vi "SendPanelUIReference.vi"(8 "error in (no error)":errorcluster, 10 "VI Refnum":refnum<vi>, 11 "Device in":refnum<class "Device.lvclass">) -> (0 "error out":errorcluster, 3 "Device out":refnum<class "Device.lvclass">)   [LabVIEW 2020, in "Device.lvlib" / "Device.lvclass"]
uses:
  Device.lvclass
  C:/Program Files/National Instruments/LabVIEW 2020/vi.lib/ActorFramework/Actor/Actor.lvclass
  <vilib>/ActorFramework/Actor/Actor.lvclass/Actor.ctl
  Interface/Communication Messages/Send Panel Refercence Msg/Send Panel Refercence Msg.lvclass/Send Panel Refercence Msg.ctl
  <vilib>/ActorFramework/Message Enqueuer/Message Enqueuer.lvclass/Message Enqueuer.ctl
  <vilib>/ActorFramework/Message Enqueuer/Enqueue.vi
  Interface/Communication Messages/Send Panel Refercence Msg/Send Panel Refercence Msg.lvclass
  C:/Program Files/National Instruments/LabVIEW 2020/vi.lib/ActorFramework/Message/Message.lvclass
  <vilib>/ActorFramework/Message Priority Queue/Priority Enqueue.vi
  <vilib>/ActorFramework/Actor/Actor.lvclass
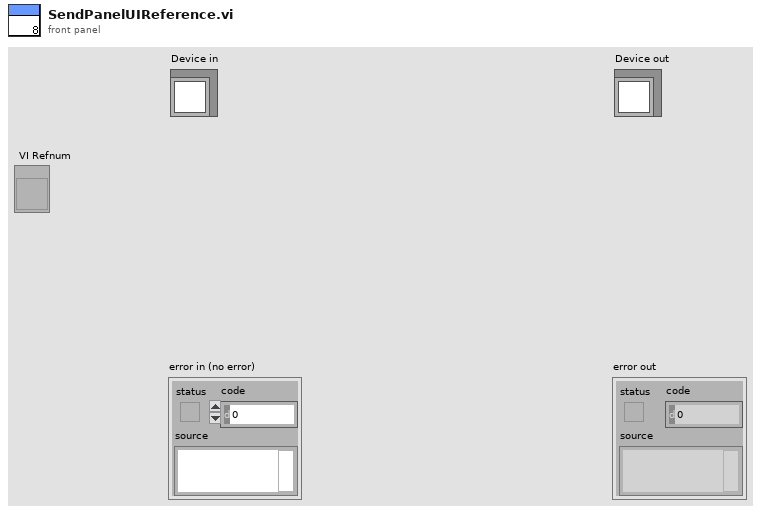
[diagram p1: front panel]
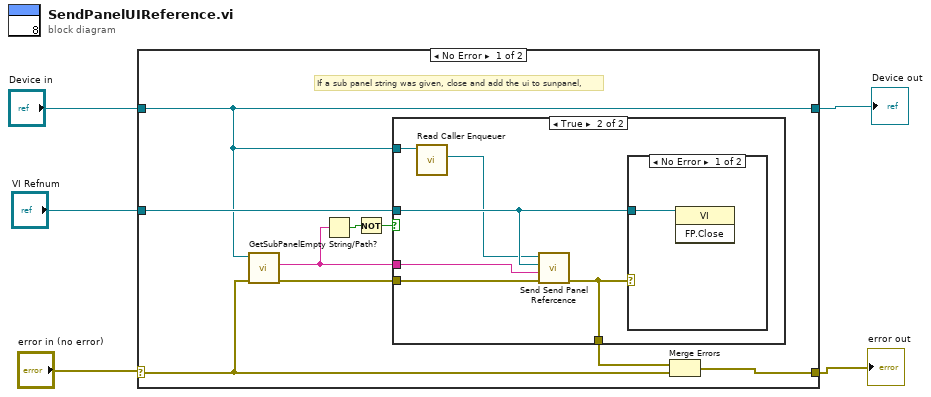
[diagram p0: block diagram]
diagram:
  n1 = case shown="No Error" "error in (no error)" {
    selector: "error in (no error)" -> [w11 w24]
    tunnel: [w14 w24] -> w2
    tunnel: [w12 w23] -> w3
    tunnel: "Device in" -> [w12 w23]
    tunnel: "VI Refnum" -> [w13 _]
    frame No Error {
      # "If a sub panel string was given, close and add the ui to sunpanel,"
      n2 = call-dynamic "GetSubPanel.vi"("error in (no error)"=w11, "Device in"=w12) -> ("error out"=w10:errorcluster, "Sub Panel"=w6:string)  [unwired: 7 in, 1 out]
      n3 = Empty String/Path?(string/path=w6) -> (empty?=w7:bool)
      n4 = Not(x=w7) -> (.not. x?=w8:bool)
      n5 = case shown="True" w8 {
        tunnel: w13 -> [_ w21]
        tunnel: w12 -> [_ w20]
        tunnel: w10 -> [w15 w19]
        tunnel: w6 -> [_ w18]
        tunnel: [w15 w16] -> w9
        frame False {
        }
        frame True {
          n6 = call <vilib>:"Read Caller Enqueuer.vi"("Actor"=w20) -> ("Caller Enqueuer"=w17:refnum<class "Message Enqueuer.lvclass">)  [unwired: 10 in]
          n7 = call "Send Send Panel Refercence.vi"("error in (no error)"=w19, "Sub Panel"=w18, "VI Refnum"=w21, "Message Enqueuer"=w17) -> ("error out"=w16:errorcluster)  [unwired: 6 in, 1 out]
          n8 = case shown="No Error" w16 {
            tunnel: w21 -> [w22 _]
            frame No Error {
              n9 = invoke class="VI" method="FP.Close"(reference=w22) -> ()  [unwired: 2 in, 3 out]
            }
            frame Error {
            }
          }
        }
      }
      n10 = Merge Errors(w9, w11) -> (w14:errorcluster)
    }
    frame Error {
    }
  }
  "error out" <- w2
  "Device out" <- w3
